vi "ASDReflectance.vi"(0 "TCP Network Connection Refnum":refnum<k5>, 7 "Collect Reflectance Spectrum":bool, 11 "error in (no error)":errorcluster) -> (4 "Header Code":i32, 6 "Error Code":i32, 8 "Reflectance Spectrum":dbl[](array[numeric]), 15 "error out":errorcluster)   [LabVIEW 2010]
panel:
  out "White Reference  Data":dbl[](array[numeric])
  out "Spectrum Data":dbl[](array[numeric])
  # "This is a Sub-VI of ASDTCPDemo."
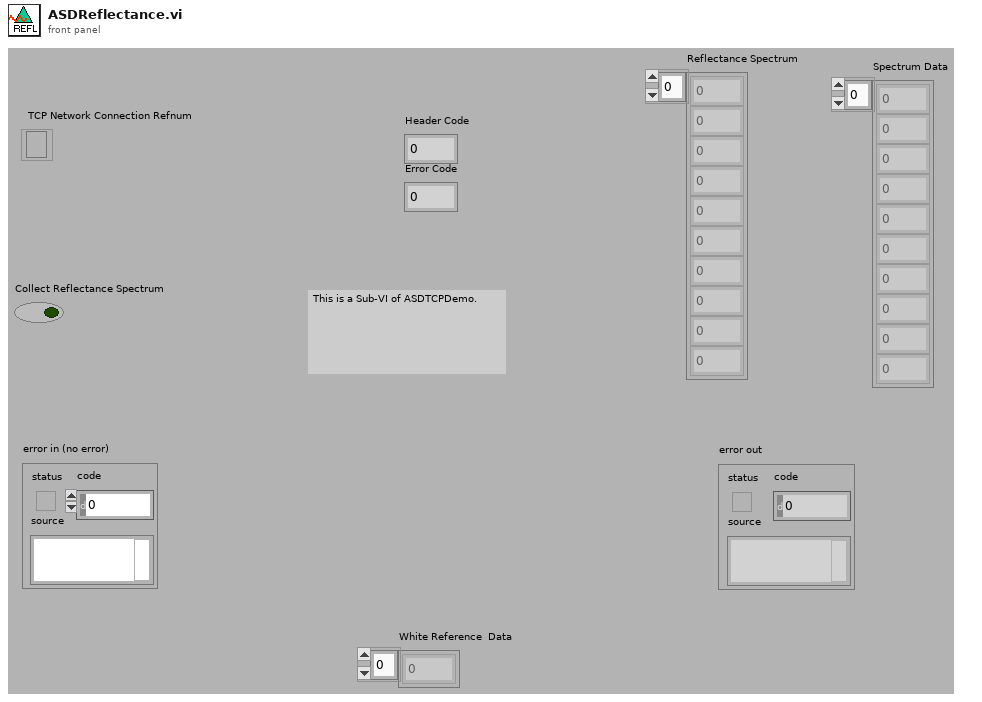
[diagram p1: front panel]
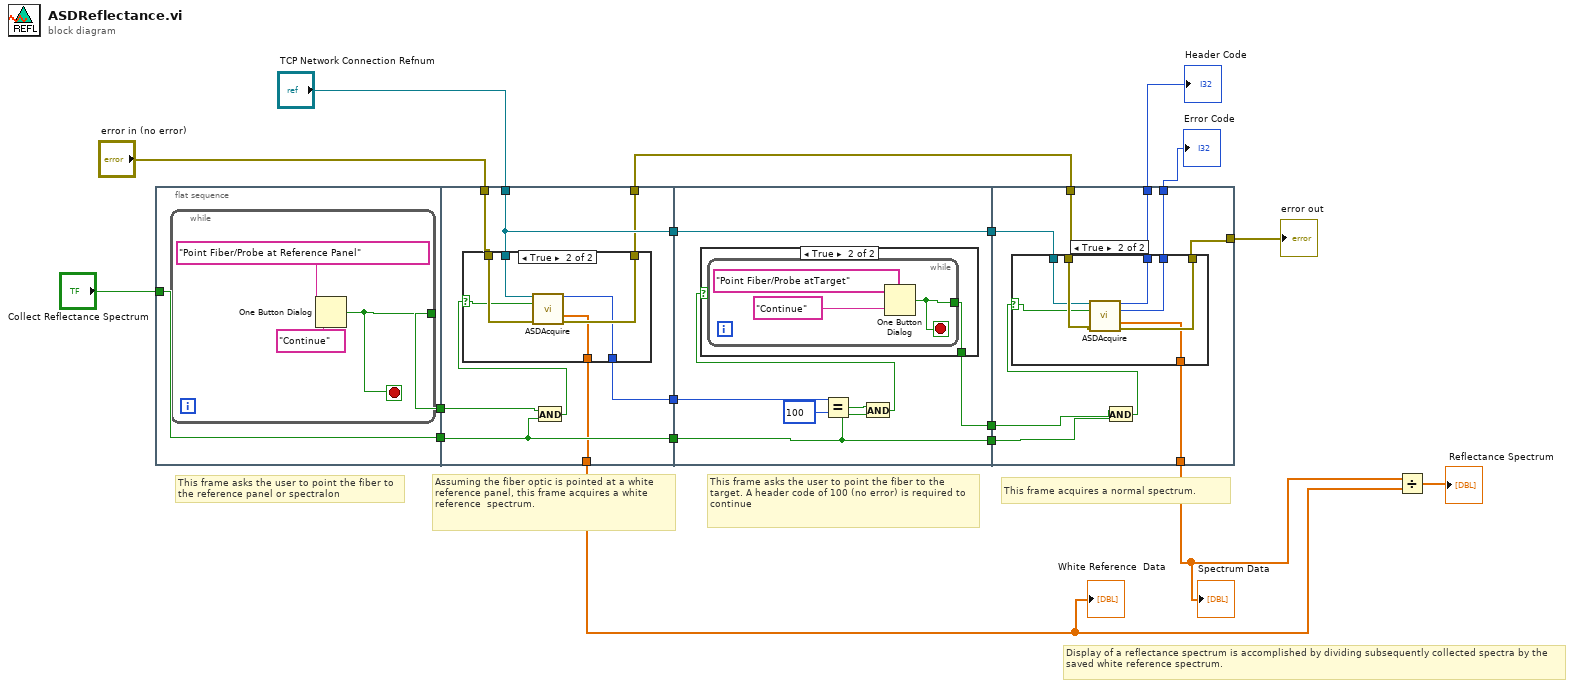
[diagram p0: block diagram]
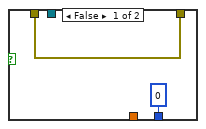
[diagram p2: hidden frame]
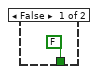
[diagram p3: hidden frame]
diagram:
  # "This frame asks the user to point the fiber to the target. A header code of 100 (no error) is required to continue"
  # "Display of a reflectance spectrum is accomplished by dividing subsequently collected spectra by the saved white reference spectrum."
  # "This frame acquires a normal spectrum."
  # "Assuming the fiber optic is pointed at a white reference panel, this frame acquires a white  reference  spectrum."
  # "This frame asks the user to point the fiber to the reference panel or spectralon"
  n1 = flat-sequence {
    tunnel: "Collect Reflectance Spectrum" -> [w20]
    tunnel: [w20] -> w17
    tunnel: [w19] -> w2
    tunnel: [w27] -> w16
    tunnel: [w24] -> w7
    tunnel: w17 -> [w29]
    tunnel: [w30] -> w15
    tunnel: [w29] -> w14
    tunnel: "error in (no error)" -> [w28]
    tunnel: "TCP Network Connection Refnum" -> [w27]
    tunnel: [w26] -> w3
    tunnel: w2 -> [w25]
    tunnel: w16 -> [w41]
    tunnel: [w41] -> w13
    tunnel: w15 -> [w44]
    tunnel: w14 -> [w42]
    tunnel: [w42] -> w12
    tunnel: [w40] -> w1
    tunnel: [w60] -> w18
    tunnel: w13 -> [w59]
    tunnel: [w58] -> w6
    tunnel: [w56] -> w9
    tunnel: [w57] -> w10
    tunnel: w12 -> [w54]
    tunnel: w3 -> [w53]
    tunnel: w1 -> [w52]
    frame #0 {
      n2 = while {
        tunnel: [w21] -> w19
        stop <- w21 stop-if-true
        n3 = One Button Dialog(message="Point Fiber/Probe at Reference Panel", button name ("OK")="Continue") -> (true=w21:bool)
      }
    }
    frame #1 {
      n4 = And(x=w25, y=w29) -> (x .and. y?=w31:bool)
      n5 = case shown="True" w31 {
        selector: w31 -> [_ w34]
        tunnel: w28 -> [w33 w39]
        tunnel: [w33 w38] -> w26
        tunnel: w27 -> [_ w37]
        tunnel: [_ w36] -> w24
        tunnel: [0 ("Header Code") w35] -> w30
        frame False {
        }
        frame True {
          n6 = call "ASDAcquire.vi"("TCP Network Connection Refnum"=w37, "Acquire"=w34, "error in (no error)"=w39) -> ("Header Code"=w35:i32, "Spectrum Data"=w36:sgl[], "error out"=w38:errorcluster)  [unwired: 9 in, 1 out]
        }
      }
    }
    frame #2 {
      n7 = Equal?(x=w44, y=100) -> (x = y?=w46:bool)
      n8 = And(x=w46, y=w42) -> (x .and. y?=w43:bool)
      n9 = case shown="True" w43 {
        tunnel: [FALSE ("true") w48] -> w40
        frame False {
        }
        frame True {
          n10 = while {
            tunnel: [w49] -> w48
            stop <- w49 stop-if-true
            n11 = One Button Dialog(message="Point Fiber/Probe atTarget", button name ("OK")="Continue") -> (true=w49:bool)
          }
        }
      }
    }
    frame #3 {
      n12 = And(x=w52, y=w54) -> (x .and. y?=w55:bool)
      n13 = case shown="True" w55 {
        selector: w55 -> [_ w62]
        tunnel: [w61 w68] -> w60
        tunnel: w53 -> [w61 w67]
        tunnel: w59 -> [_ w66]
        tunnel: [_ w65] -> w58
        tunnel: [_ w64] -> w56
        tunnel: [_ w63] -> w57
        frame False {
        }
        frame True {
          n14 = call "ASDAcquire.vi"("TCP Network Connection Refnum"=w66, "Acquire"=w62, "error in (no error)"=w67) -> ("Header Code"=w64:i32, "Error Code"=w63:i32, "Spectrum Data"=w65:sgl[], "error out"=w68:errorcluster)  [unwired: 9 in]
        }
      }
    }
  }
  n15 = Divide(x=w6, y=w7) -> (x/y=→"Reflectance Spectrum":sgl[])
  "error out" <- w18
  "Header Code" <- w9
  "Error Code" <- w10
  "Spectrum Data" <- w6
  "White Reference  Data" <- w7
